vi "Teleop.vi"(10 "Match Info":T1={"Autonomous Elapsed Seconds"=0.0, "TeleOp Elapsed Seconds"=0.0, "Disabled Elapsed Seconds"=0.0, "Visited Autonomous"=FALSE, "Visited TeleOp"=FALSE, "Visited Disabled"=FALSE, "Autonomous Settings"={"Autonomous Style"=enum."Independent", "VI Refnum"=refnum}}, 11 "Call Context":T2) -> ()   [LabVIEW 2016]
doc: "This VI is called for each TeleOp packet received from the DS where the robot is not disabled. It is often used to read from the joysticks and update I/O or to update setpoints for timed control loops. It should complete and return within 20 milliseconds or it may miss DS packets."
uses:
  <vilib>/Rock Robotics/WPI/DriverStation/WPI_DriverStationDerivedRobotMode.ctl
  <vilib>/Rock Robotics/WPI/DriverStation/WPI_DriverStationMatch Info.ctl
  <vilib>/Rock Robotics/WPI/Solenoid/WPI_SolenoidValue.ctl
  <vilib>/Rock Robotics/WPI/Utilities/WPI_GetSetVariantRefNum.vi
  <vilib>/Rock Robotics/WPI/Joystick/WPI_JoystickArcadeMapping.vi
  <vilib>/Rock Robotics/WPI/Solenoid/WPI_SolenoidSetEnum.vi
panel:
  out "Buttons":bool[](array[boolean])
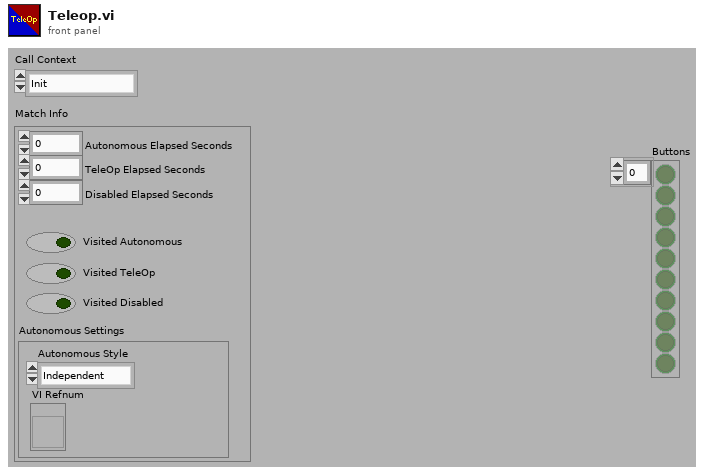
[diagram p1: front panel]
types:
  T1 = typedef "WPI_DriverStationMatch Info.ctl" = cluster{"Autonomous Elapsed Seconds":dbl, "TeleOp Elapsed Seconds":dbl, "Disabled Elapsed Seconds":dbl, "Visited Autonomous":bool, "Visited TeleOp":bool, "Visited Disabled":bool, "Autonomous Settings":cluster{"Autonomous Style":enum16{"Iterative", "Independent"}, "VI Refnum":refnum<vi>}}
  T2 = typedef "WPI_DriverStationDerivedRobotMode.ctl" = enum16{"Init", "Execute", "Stop"}
  T3 = typedef "WPI_SolenoidValue.ctl" = enum16{"Off", "On", "Forward", "Reverse"}
  T4 = typedef "WPI_JoystickDevRef.ctl" = cluster{"Device":T5}
  T5 = typedef "WPI_JoystickDeviceEnum.ctl" = enum16{"USB 0", "USB 1", "USB 2", "USB 3", "USB 4", "USB 5"}
  T6 = typedef "WPI_MotorControlDeviceRef.ctl" = cluster{"DeviceStatus":errorcluster, "Type":T7, "PWM":cluster{"PWM Channel":T8, "DeadBand":T9}, "CAN":cluster{"Device Number":u8, "SetOutput VI Ref":variant, "GetOutput VI Ref":variant, "Enable VI Ref":variant, "Disable VI Ref":variant, "Data":variant}, "Invert":bool}
  T7 = typedef "WPI_MotorControlType.ctl" = enum16{"PWM", "CAN"}
  T8 = typedef "FPGA_DIOPWMChannel.ctl" = enum8{"PWM 0", "PWM 1", "PWM 2", "PWM 3", "PWM 4", "PWM 5", "PWM 6", "PWM 7", "PWM 8", "PWM 9", "PWM MXP 0", "PWM MXP 1", "PWM MXP 2", "PWM MXP 3", "PWM MXP 4", "PWM MXP 5", "PWM MXP 6", "PWM MXP 7", "PWM MXP 8", "PWM MXP 9", "Invalid"}
  T9 = typedef "WPI_PWMDeadband.ctl" = cluster{"Name":string, "maxPositivePwm":i32, "minPositivePwm":i32, "centerPwm":i32, "maxNegativePwm":i32, "minNegativePwm":i32, "angularRange":u16}
  T10 = typedef "WPI_SolenoidDevRef.ctl" = cluster{"DevStatus":errorcluster, "Pneumatics Control Module":u8, "Forward Solenoid Channel":T11, "Reverse Solenoid Channel":T11}
  T11 = typedef "WPI_SolenoidChannel.ctl" = enum8{"Solenoid 0", "Solenoid 1", "Solenoid 2", "Solenoid 3", "Solenoid 4", "Solenoid 5", "Solenoid 6", "Solenoid 7", "Invalid"}
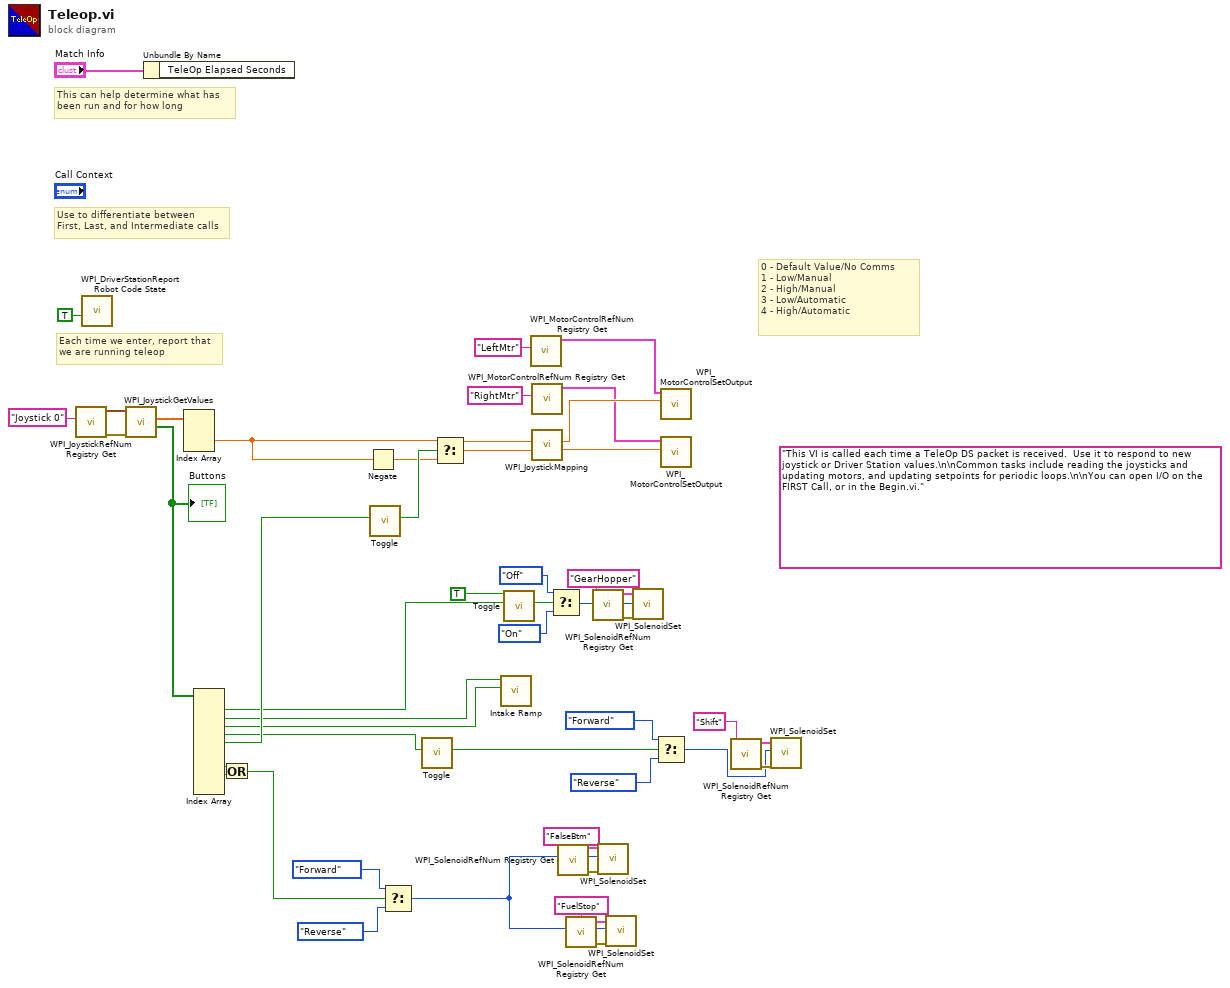
[diagram p0: block diagram]
diagram:
  (unwired) "This VI is called each time a TeleOp DS packet is received.  Use it to respond to new joystick or Driver Station values.\n\nCommon tasks include reading the joysticks and updating motors, and updating setpoints for periodic loops.\n\nYou can open I/O on the FIRST Call, or in the Begin.vi."
  # "0 - Default Value/No Comms\n1 - Low/Manual\n2 - High/Manual\n3 - Low/Automatic\n4 - High/Automatic"
  # "Each time we enter, report that\nwe are running teleop"
  # "Use to differentiate between\nFirst, Last, and Intermediate calls"
  # "This can help determine what has\nbeen run and for how long"
  n1 = call <vilib>:"WPI_JoystickRefNum Registry Get.vi"("refnum name"="Joystick 0") -> ("error out"=w34:errorcluster, "JoystickDevRef"=w48:T4)  [unwired: 1 in, 8 out]
  n2 = call <vilib>:"WPI_DriverStationReport Robot Code State.vi"("TeleOp"=TRUE ("Autonomous")) -> ()  [unwired: 10 in, 1 out]
  n3 = call <vilib>:"WPI_JoystickGetValues.vi"("error in (no error)"=w34, "JoystickDevRef"=w48) -> ("Buttons"=w45:bool[], "Axes"=w46:dbl[])  [unwired: 5 in, 3 out]
  "Buttons" <- w45
  n4 = Unbundle By Name("Match Info") -> ()  [unwired: 1 out]
  n5 = Index Array(array=w46) -> (element #1=w14:dbl, element #2=w15:dbl)  [unwired: 3 in, 1 out]
  n6 = Index Array(array=w45) -> (element #1=w38:bool, element #2=w17:bool, element #3=w16:bool, element #4=w3:bool, element #5=w42:bool, element #8=w36:bool, element #9=w37:bool)  [unwired: 11 in, 4 out]
  n7 = Or(x=w36, y=w37) -> (x .or. y?=w13:bool)
  n8 = Negate(x=w15) -> (-x=w40:dbl)
  n9 = call "Toggle.vi"("Input"=w42) -> ("Output"=w41:bool)  [unwired: 10 in]
  n10 = Select(t=WPI_SolenoidValue."Forward" ("Value"), s=w13, f=WPI_SolenoidValue."Reverse" ("Value")) -> (s? t:f=w24:T3)
  n11 = call "Toggle.vi"("Input"=w3) -> ("Output"=w4:bool)  [unwired: 10 in]
  n12 = Select(t=w15, s=w41, f=w40) -> (s? t:f=w35:dbl)
  n13 = call "Intake Ramp.vi"("Intake"=w16, "Outtake"=w17) -> ()  [unwired: 10 in]
  n14 = call "Toggle.vi"("Control"=TRUE, "Input"=w38) -> ("Output"=w30:bool)  [unwired: 9 in]
  n15 = call <vilib>:"WPI_MotorControlRefNum Registry Get.vi"("refnum name"="LeftMtr") -> ("MotorControlDevRef"=w2:T6)  [unwired: 9 in, 1 out]
  n16 = call <vilib>:"WPI_MotorControlRefNum Registry Get.vi"("refnum name"="RightMtr") -> ("MotorControlDevRef"=w1:T6)  [unwired: 9 in, 1 out]
  n17 = call-poly <vilib>:"WPI_JoystickMapping.vi"("Y axis value"=w35, "X axis value"=w14) -> ("Right Motor Value"=w11:dbl, "Left Motor Value"=w12:dbl)  [unwired: 8 in]
  n18 = Select(t=WPI_SolenoidValue."Off" ("Value"), s=w30, f=WPI_SolenoidValue."On" ("Value")) -> (s? t:f=w27:T3)
  n19 = call <vilib>:"WPI_SolenoidRefNum Registry Get.vi"("refnum name"="FalseBtm") -> ("error out"=w19:errorcluster, "SolenoidDevRef"=w20:T10)  [unwired: 9 in]
  n20 = call <vilib>:"WPI_SolenoidRefNum Registry Get.vi"("refnum name"="FuelStop") -> ("error out"=w18:errorcluster, "SolenoidDevRef"=w21:T10)  [unwired: 9 in]
  n21 = call <vilib>:"WPI_SolenoidRefNum Registry Get.vi"("refnum name"="GearHopper") -> ("error out"=w32:errorcluster, "SolenoidDevRef"=w31:T10)  [unwired: 9 in]
  n22 = call-poly <vilib>:"WPI_SolenoidSet.vi"("error in (no error)"=w19, "Value"=w24, "SolenoidDevRef"=w20) -> ()  [unwired: 7 in, 2 out]
  n23 = call-poly <vilib>:"WPI_SolenoidSet.vi"("error in (no error)"=w18, "Value"=w24, "SolenoidDevRef"=w21) -> ()  [unwired: 7 in, 2 out]
  n24 = call-poly <vilib>:"WPI_SolenoidSet.vi"("error in (no error)"=w32, "Value"=w27, "SolenoidDevRef"=w31) -> ()  [unwired: 7 in, 2 out]
  n25 = Select(t=WPI_SolenoidValue."Forward" ("Value"), s=w4, f=WPI_SolenoidValue."Reverse" ("Value")) -> (s? t:f=w5:T3)
  n26 = call <vilib>:"WPI_MotorControlSetOutput.vi"("Output"=w12, "MotorControlDevRef"=w2) -> ()  [unwired: 7 in, 3 out]
  n27 = call <vilib>:"WPI_MotorControlSetOutput.vi"("Output"=w11, "MotorControlDevRef"=w1) -> ()  [unwired: 7 in, 3 out]
  n28 = call <vilib>:"WPI_SolenoidRefNum Registry Get.vi"("refnum name"="Shift") -> ("error out"=w9:errorcluster, "SolenoidDevRef"=w10:T10)  [unwired: 9 in]
  n29 = call-poly <vilib>:"WPI_SolenoidSet.vi"("error in (no error)"=w9, "Value"=w5, "SolenoidDevRef"=w10) -> ()  [unwired: 7 in, 2 out]
